vi "Format_html_report.vi"(9 "Sample Information":T1 {"Session_list"."Instrument" items=["Unknown", "Phillips SEM IRC", "JEOL 7000F EML_MFC", "MXRD MFC", "JEOL_EPMA"]}, 10 "Sample_data_base":path, 11 "Table in":refnum<vi>) -> (3 "String":string)   [LabVIEW 2011]
uses:
  Sample_top_level.ctl
  Sample_Session_info.ctl
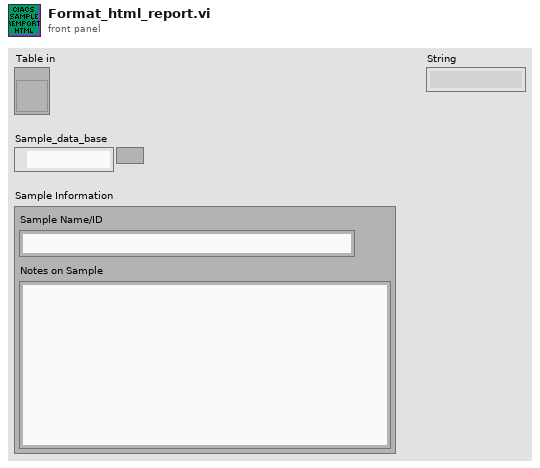
[diagram p1: front panel]
types:
  T1 = typedef "Sample_top_level.ctl" = cluster{"Sample Name/ID":string, "Notes on Sample":string, "Session_list":T2[]}
  T2 = typedef "Sample_Session_info.ctl" = cluster{"Instrument":u16, "Session_data_base":path, "Session Name/ID":string}
  T3 = typedef "cm2nm_sample_set.ctl" = cluster{"CollectionOfPoints":T4[], "Instrument":T5, "CollectionFile":path, "Session Name/ID":string, "SessionNotes":string}
  T4 = typedef "cm2nm_coordinate_information_v2.ctl" = cluster{"MetaDataFile":path, "X":dbl, "Y":dbl, "Z":dbl, "Group":i32, "Rotation":dbl[unit], "Fiducial":bool, "Magnification":dbl, "Working_Distance":dbl, "Notes":string, "Location Name/ID":string, "OtherRelatedDataFiles":cluster{"Type of File":string, "FileName":path}[], "Available":bool}
  T5 = typedef "Instrument_type_enum_v2.ctl" = enum16{"Unknown", "Philips FEI SEM IRC", "JEOL 7000F EML_MFC", "MXRD MFC", "JEOL_EPMA"}
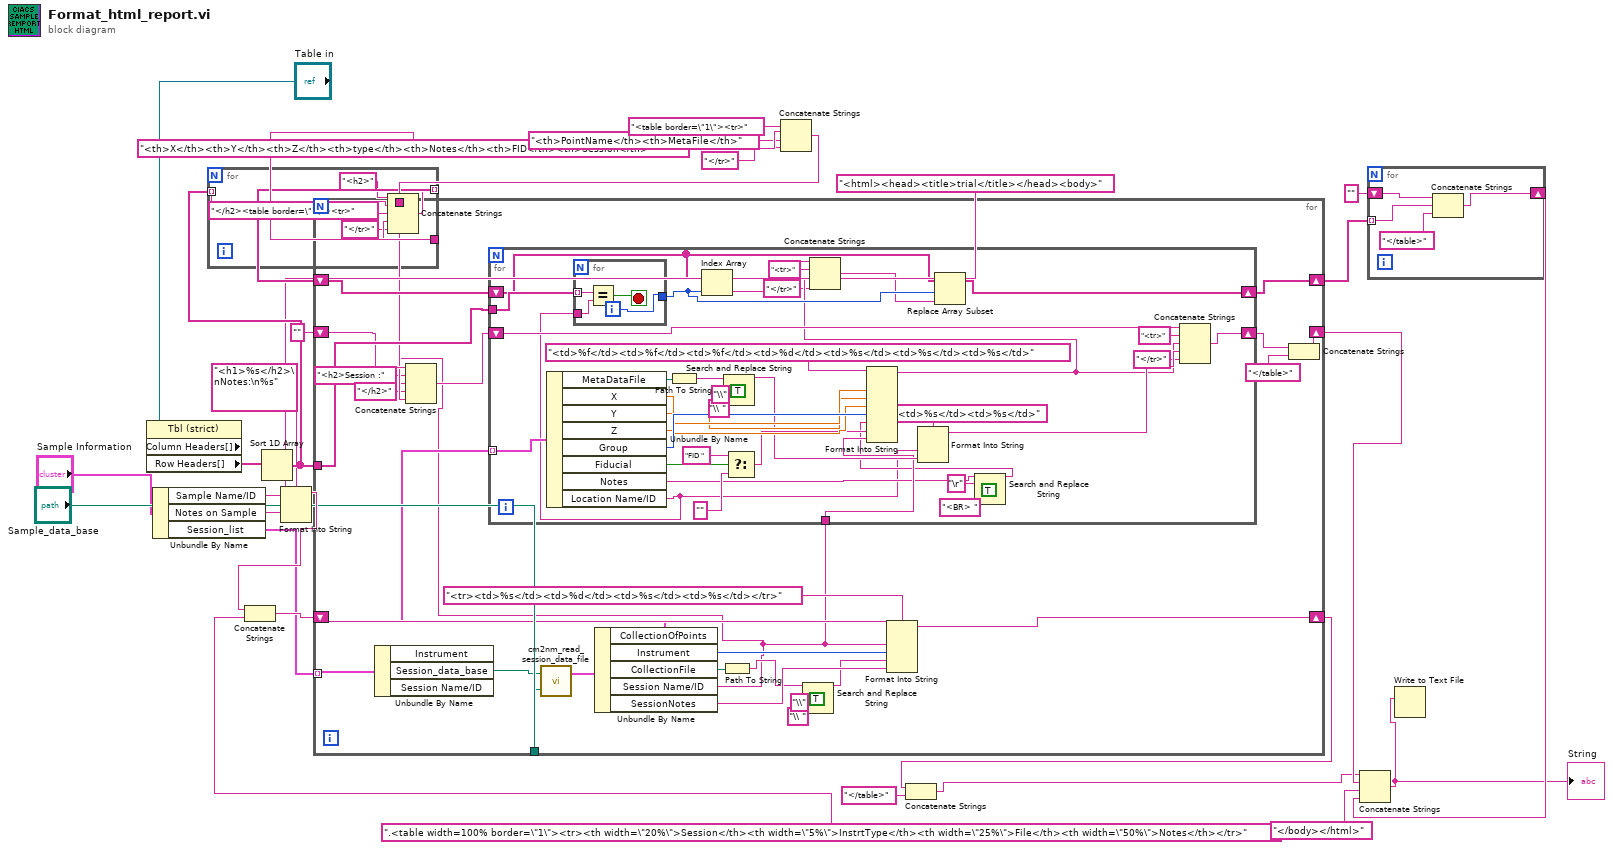
[diagram p0: block diagram]
diagram:
  w22 = "<th>X</th><th>Y</th><th>Z</th><th>type</th><th>Notes</th><th>FID</th><th>Session</th>" ("format string")
  n1 = property on="Property Node" class="Tbl (strict)" props=["Column Headers[]", "Row Headers[]"](reference="Table in") -> ("Row Headers[]"=w3:string[])  [unwired: 1 in, 3 out]
  n2 = Unbundle By Name("Sample Information") -> ("Sample Name/ID"=w6:string, "Notes on Sample"=w7:string, "Session_list"=w4:T2[])
  n3 = Sort 1D Array(array=w3) -> (sorted array=w20:string[])
  n4 = for {
    tunnel: w20 -> [w35] mode=indexing
    tunnel: [w32] -> w21 mode=indexing
    tunnel: w22 -> [w31]
    n5 = Concatenate Strings("<h2>" ("string"), w35, "</h2><table border=\"1\"><tr>" ("string"), w31, "</tr>" ("string")) -> (w32:string)
  }
  n6 = Format Into String(format string="<h1>%s</h2>\nNotes:\n%s", initial string="<html><head><title>trial</title></head><body>", w6, w7) -> (resulting string=w15:string)  [unwired: 1 in, 1 out]
  n7 = Concatenate Strings(w15, ".<table width=100% border=\"1\"><tr><th width=\"20%\">Session</th><th width=\"5%\">InstrtType</th><th width=\"25%\">File</th><th width=\"50%\">Notes</th></tr>" ("initial string")) -> (w14:string)
  n8 = Concatenate Strings("<table border=\"1\"><tr>" ("string"), w22, "<th>PointName</th><th>MetaFile</th>" ("format string"), "</tr>" ("string")) -> (w27:string)
  n9 = for {
    tunnel: w4 -> [w63] mode=indexing
    tunnel: w20 -> [w46]
    tunnel: "Sample_data_base" -> [w59]
    shift-right: [w54] -> w10
    shift-left: w14 -> [w55]
    shift-right: [w42] -> w25
    shift-left: "" -> [w41]
    shift-right: [w45] -> w23
    shift-left: w21 -> [w47]
    tunnel: w27 -> [w39]
    n10 = Unbundle By Name(w63) -> ("Session_data_base"=w62:path)  [unwired: 2 out]
    n11 = call "cm2nm_read_session_data_file.vi"("TopLevelDataFilePath"=w59, "Session_data_base"=w62) -> ("Session Information"=w61:T3)  [unwired: 1 in]
    n12 = Unbundle By Name(w61) -> ("CollectionOfPoints"=w48:T4[], "Instrument"=w57:T5, "CollectionFile"=w60:path, "Session Name/ID"=w37:string, "SessionNotes"=w56:string)
    n13 = Concatenate Strings(w41, "<h2>Session :" ("string"), w37, "</h2>" ("string"), w39) -> (w40:string)
    n14 = for {
      tunnel: w48 -> [w101] mode=indexing
      shift-right: [w80] -> w43
      shift-left: w40 -> [w84]
      tunnel: w37 -> [w79]
      shift-right: [w64] -> w45
      shift-left: w47 -> [w70]
      tunnel: w46 -> [w73]
      n15 = Unbundle By Name(w101) -> ("MetaDataFile"=w100:path, "X"=w93:dbl, "Y"=w92:dbl, "Z"=w91:dbl, "Group"=w94:i32, "Fiducial"=w90:bool, "Notes"=w76:string, "Location Name/ID"=w72:string)
      n16 = for {
        tunnel: w73 -> [w105] mode=indexing
        tunnel: w72 -> [w104]
        tunnel: [w102] -> w71
        i -> [w102]
        stop <- w103 stop-if-true
        n17 = Equal?(x=w105, y=w104) -> (x = y?=w103:bool)
      }
      n18 = Path To String(path=w100) -> (string=w96:string)
      n19 = Index Array(array=w70, index=w71) -> (element=w66:string)
      n20 = Search and Replace String(replace all?=TRUE ("replace all? (F)"), input string=w96, search string="\\", replace string="\\ " ("replace string (\"\")")) -> (result string=w85:string)  [unwired: 4 in, 3 out]
      n21 = Select(t="FID " ("replace string (\"\")"), s=w90, f="" ("replace string (\"\")")) -> (s? t:f=w89:string)
      n22 = Format Into String(format string="<td>%s</td><td>%s</td>", w72, w85) -> (resulting string=w82:string)  [unwired: 2 in, 1 out]
      n23 = Search and Replace String(replace all?=TRUE ("replace all? (F)"), input string=w76, search string="\r", replace string="<BR> " ("replace string (\"\")")) -> (result string=w75:string)  [unwired: 4 in, 3 out]
      n24 = Format Into String(format string="<td>%f</td><td>%f</td><td>%f</td><td>%d</td><td>%s</td><td>%s</td><td>%s</td>", w93, w92, w91, w94, w75, w89, w79) -> (resulting string=w68:string)  [unwired: 2 in, 1 out]
      n25 = Concatenate Strings(w66, "<tr>" ("string"), w68, "</tr>" ("string")) -> (w65:string)
      n26 = Replace Array Subset(array=w70, new element=w65, index=w71) -> (w64:string[])
      n27 = Concatenate Strings(w84, "<tr>" ("string"), w68, w82, "</tr>" ("string")) -> (w80:string)
    }
    n28 = Path To String(path=w60) -> (string=w53:string)
    n29 = Search and Replace String(replace all?=TRUE ("replace all? (F)"), input string=w53, search string="\\", replace string="\\ " ("replace string (\"\")")) -> (result string=w52:string)  [unwired: 4 in, 3 out]
    n30 = Format Into String(format string="<tr><td>%s</td><td>%d</td><td>%s</td><td>%s</td></tr>", initial string=w55, w37, w57, w52, w56) -> (resulting string=w54:string)  [unwired: 1 in, 1 out]
    n31 = Concatenate Strings(w43, "</table>" ("string")) -> (w42:string)
  }
  n32 = Concatenate Strings(w10, "</table>" ("string")) -> (w18:string)
  n33 = for {
    tunnel: w23 -> [w108] mode=indexing
    shift-right: [w107] -> w24
    shift-left: "" -> [w109]
    n34 = Concatenate Strings(w109, w108, "</table>" ("string")) -> (w107:string)
  }
  n35 = Concatenate Strings(w18, w25, "</body></html>" ("string"), w24) -> (w19:string)
  "String" <- w19
  n36 = Write to Text File(text=w19) -> ()  [unwired: 3 in, 3 out]
